vi "Do.vi"(8 "error in (no error)":errorcluster, 10 "Actor in":refnum<class "Actor.lvclass">, 11 "Set Output Voltage Msg":refnum<class "Set Output Voltage Msg.lvclass">) -> (0 "error out":errorcluster, 2 "Actor out":refnum<class "Actor.lvclass">)   [LabVIEW 2016, in "BNT_DAQmx.lvlib" / "Set Output Voltage Msg.lvclass"]
doc: "This VI delivers the message to the actor by calling the appropriate method(s) on the actor."
uses:
  Set Output Voltage Msg.lvclass
  <vilib>/ActorFramework/Actor/Actor.lvclass
  C:/User/Brand/LVP/TASCA/UTCS/Packages/CSPP_Core/Actors/CS++PVMonitor Messages/CS++PVUpdate Msg/CS++PVUpdate Msg.lvclass
  BNT_DAQmx-MCSV/BNT_DAQmx-MCSV.lvclass
  C:/Program Files (x86)/National Instruments/LabVIEW 2016/vi.lib/ActorFramework/Actor/Actor.lvclass
  Set Output Voltage Msg.lvclass/Set Output Voltage Msg.ctl
  BNT_DAQmx-MCSV/BNT_DAQmx-MCSV.lvclass/BNT_DAQmx-MCSV.ctl
  CSPP_Core/Actors/CS++PVMonitor Messages/CS++PVUpdate Msg/CS++PVUpdate Msg.lvclass/CS++PVUpdate Msg.ctl
  CSPP_Core/Classes/CS++ProcessVariables/ProcessVariable/PV.lvclass/PV.ctl
  CSPP_Core/Classes/CS++ProcessVariables/ProcessVariable/PV.lvclass
  CSPP_Core/Actors/CS++PVMonitor Messages/CS++PVUpdate Msg/CS++PVUpdate Msg.lvclass
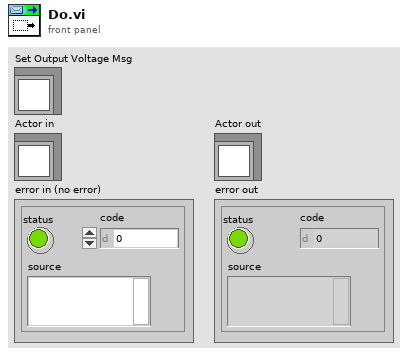
[diagram p1: front panel]
types:
  T1 = cluster{"Voltage":dbl[unit], "index of element":i32}
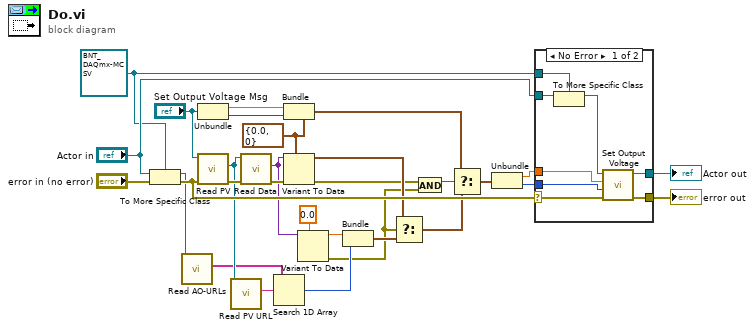
[diagram p0: block diagram]
diagram:
  w23 = cluster{"Voltage":dbl[unit], "Channel":i32} {"Voltage"=0.0, "Channel"=0} ("Type")
  w26 = refnum<class "BNT_DAQmx-MCSV.lvclass"> refnum ("Actor in")
  n1 = To More Specific Class(target class=w26, reference="Actor in", error in="error in (no error)") -> (specific class reference=w2:refnum<class "BNT_DAQmx-MCSV.lvclass">, error out=w19:errorcluster)
  n2 = call "Read AO-URLs.vi"("BNT_DAQmx-MCSV in"=w2) -> ("AO-URLs"=w1:string[])  [unwired: 9 in, 1 out]
  n3 = Unbundle ("Pre-Unbundler")("Set Output Voltage Msg") -> (w16:dbl[unit], w15:i32)
  n4 = call "Read PV.vi"("error in (no error)"=w19, "CS++PVUpdate Msg in"="Set Output Voltage Msg") -> ("error out"=w25:errorcluster, "PV"=w10:refnum<class "PV.lvclass">)  [unwired: 7 in, 1 out]
  n5 = call "Read PV URL.vi"("PV in"=w10) -> ("PV URL"=w12:string)  [unwired: 8 in, 2 out]
  n6 = call "Read Data.vi"("error in (no error)"=w25, "PV in"=w10) -> ("error out"=w22:errorcluster, "Data"=w8:variant)  [unwired: 7 in, 1 out]
  n7 = Search 1D Array(1D array=w1, element=w12) -> (index of element=w13:i32)  [unwired: 1 in]
  n8 = Bundle ("Pre-Bundler")(cluster=w23, "Voltage"=w16, "Channel"=w15) -> (w24:cluster{"Voltage":dbl[unit], "Channel":i32})
  n9 = Variant To Data(error in=w22, type=w23, Variant=w8) -> (data=w7:cluster{"Voltage":dbl[unit], "Channel":i32}, error out=w4:errorcluster)
  n10 = Variant To Data(type=dbl[unit] 0.0 ("Voltage"), Variant=w8) -> (data=w11:dbl[unit], error out=w5:errorcluster)  [unwired: 1 in]
  n11 = Bundle ("Pre-Bundler")("Voltage"=w11, "index of element"=w13) -> (w14:T1)  [unwired: 1 in]
  n12 = Select ("MainSelect")(t=w7, s=w5, f=w14) -> (s? t:f=w6:T1)
  n13 = And(x=w4, y=w5) -> (x .and. y?=w3:bool)
  n14 = Select ("MainSelect")(t=w24, s=w3, f=w6) -> (s? t:f=w21:T1)
  n15 = Unbundle ("Main-Unbundler")(w21) -> ("Voltage"=w18:dbl[unit], "index of element"=w17:i32)
  n16 = case shown="No Error" w19 {
    selector: w19 -> [w36 w40]
    tunnel: [w38 w40] -> w29
    tunnel: [w37 w39] -> w28
    tunnel: "Actor in" -> [w35 w39]
    tunnel: w26 -> [w34 _]
    tunnel: w18 -> [w32 _]
    tunnel: w17 -> [w31 _]
    frame No Error {
      n17 = To More Specific Class(target class=w34, reference=w35) -> (specific class reference=w33:refnum<class "BNT_DAQmx-MCSV.lvclass">)  [unwired: 1 in, 1 out]
      n18 = call "Set Output Voltage.vi"("Error In"=w36, "Channel"=w31, "Voltage"=w32, "BNT_DAQmx-MCSV in"=w33) -> ("Error Out"=w38:errorcluster, "BNT_DAQmx-MCSV out"=w37:refnum<class "BNT_DAQmx-MCSV.lvclass">)  [unwired: 6 in]
    }
    frame Error {
    }
  }
  "error out" <- w29
  "Actor out" <- w28
